vi "Save New Channel Settings.vi"(10 "New Montage Name":string, 11 "EEG Channels":T1 {"16 EEG Channels"."Channel No" step=1}) -> ()   [LabVIEW 2016, in "Settings Editor.lvlib"]
uses:
  Settings Editor.lvlib
  CML Shared/EEG Channel Settings.ctl
  <vilib>/Utility/xml.llb/Write to XML File(string).vi
  CML Shared/CML Shared.lvlib
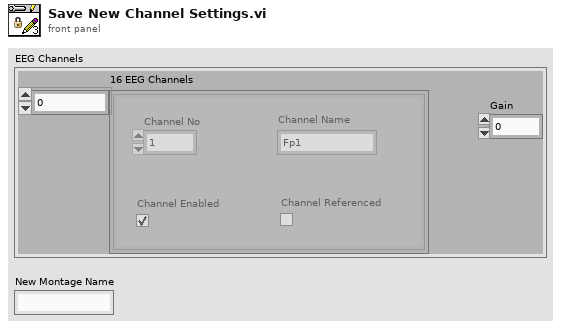
[diagram p1: front panel]
types:
  T1 = typedef "CML Shared.lvlib/EEG Channel Settings.ctl" = cluster{"16 EEG Channels":cluster{"Channel Name":string, "Channel No":u8, "Channel Enabled":bool, "Channel Referenced":bool}[], "Gain":u8}
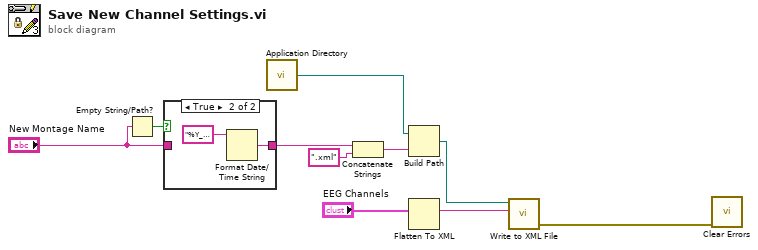
[diagram p0: block diagram]
diagram:
  n1 = Empty String/Path?(string/path="New Montage Name") -> (empty?=w3:bool)
  n2 = case shown="True" w3 {
    tunnel: [w11 w12] -> w4
    tunnel: "New Montage Name" -> [w11 _]
    frame False {
    }
    frame True {
      n3 = Format Date/Time String(time format string (%c)="%Y_%m_%d_%H_%M_%S") -> (date/time string=w12:string)  [unwired: 2 in]
    }
  }
  n4 = call <vilib>:"Application Directory.vi"() -> ("Application Directory"=w2:path)
  n5 = Concatenate Strings(w4, ".xml" ("string")) -> (w7:string)
  n6 = Build Path(base path=w2, name or relative path=w7) -> (appended path=w9:path)
  n7 = Flatten To XML(anything="EEG Channels") -> (xml string=w8:string)
  n8 = call-poly <vilib>:"Write to XML File.vi"("XML Input"=w8, "XML File Path"=w9) -> ("error out"=w1:errorcluster)  [unwired: 7 in, 2 out]
  n9 = call <vilib>:"Clear Errors.vi"("error in (no error)"=w1) -> ()  [unwired: 5 in, 2 out]
